vi "Hungry.vi"(8 "error in (no error)":errorcluster, 10 "Philosopher ID":i32, 11 "Table in":refnum<class "Table.lvclass">) -> (0 "error out":errorcluster, 3 "Table out":refnum<class "Table.lvclass">)   [LabVIEW 2023, in "Table.lvlib" / "Table.lvclass"]
uses:
  Table.lvclass
  Hungry.ctl
  Table.lvclass/Table.ctl
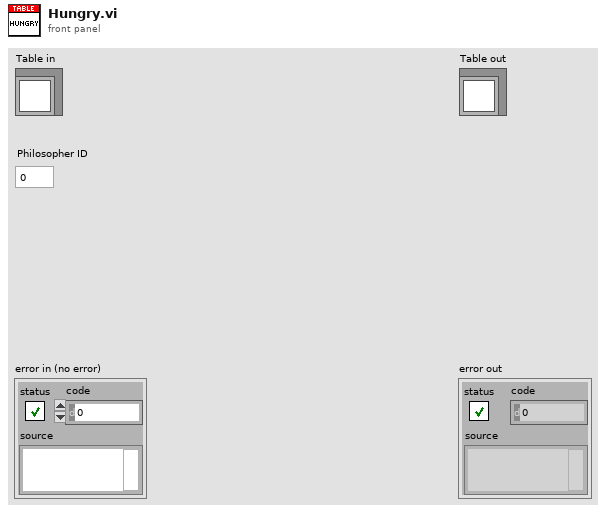
[diagram p1: front panel]
types:
  T1 = typedef "Table.lvlib/Table.lvclass/Hungry.ctl" = enum16{"NO", "YES"}
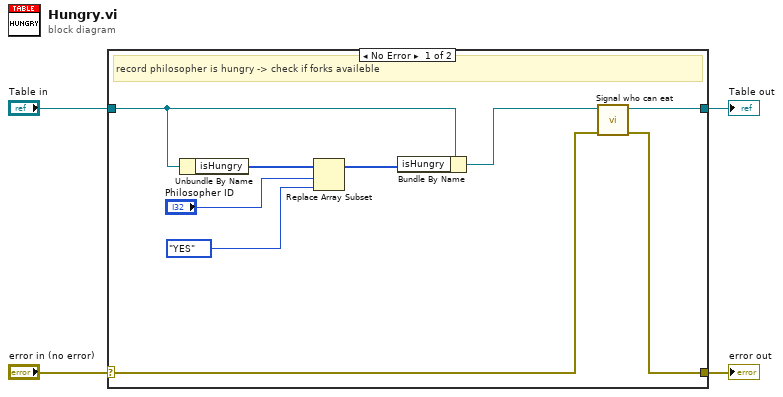
[diagram p0: block diagram]
diagram:
  n1 = case shown="No Error" "error in (no error)" {
    selector: "error in (no error)" -> [w6 w15]
    tunnel: [w5 w15] -> w3
    tunnel: [w7 w14] -> w1
    tunnel: "Table in" -> [w9 w14]
    frame No Error {
      # "record philosopher is hungry -> check if forks availeble"
      n2 = Unbundle By Name(w9) -> ("isHungry"=w13:T1[])
      n3 = Replace Array Subset(array=w13, new element=Hungry."YES" ("new element/subarray"), index="Philosopher ID") -> (w10:T1[])
      n4 = Bundle By Name(cluster=w9, "isHungry"=w10) -> (w8:refnum<class "Table.lvclass">)
      n5 = call-dynamic "Signal who can eat.vi"("error in (no error)"=w6, "Table in"=w8) -> ("error out"=w5:errorcluster, "Table out"=w7:refnum<class "Table.lvclass">)  [unwired: 8 in]
    }
    frame Error {
    }
  }
  "error out" <- w3
  "Table out" <- w1
